vi "NA.vi"() -> ()   [LabVIEW 2020]
uses:
  <instrlib>/Agilent ENA Series/Agilent ENA Series.lvlib
panel:
  out "실수값 [dB]":dbl
  out "주파수 [MHz]":dbl
  out "읽어온 데이터":string[][](table)
  in  "s2p 저장":bool caption="빈 버튼"
  in  "파일명":string
  in  "파일명":string
  in  "저장경로":path
  in  "이미지 저장":bool caption="빈 버튼"
  in  "Reset":bool
  in  "라디오 버튼":enum32{"Center / Span", "Start / Stop"}(radio)
  in  "Stop [MHz]":dbl
  in  "Start [MHz]":dbl
  in  "Span [MHz]":dbl=2000.0
  in  "Center [MHz]":dbl=5000.0
  in  "Value Graticule Line (0.0)":dbl format="%^.2e"
  in  "Data Format":u16(ring) items=["Logarithmic Magnitude", "Phase", "Group Delay", "Smith Chart  Linear (Lin/Phase)", "Smith Chart  Logarithmic (Log/Phase)", "Smith Chart  Complex (Real/Imag)", "Smith Chart  Impedance (R+jX)", "Smith Chart  Admittance (G+jB)", "Polar Format (Linear)", "Polar Format (Logarithmic)", "Polar Format (Re/Im)", "Linear Magnitude", "SWR", "Real", "Imaginary", "Epanded Phase", "Positive Phase"]
  in  "Measurement Parameters":u16(ring)=1 items=["S11"=0, "S21"=1, "S12"=4, "S22"=5, "A"=16, "B"=17, "R1"=20, "R2"=21, "AUX1"=24, "AUX2"=25]
  in  "VISA 리소스 이름":refnum<visa-resource-name>
  in  "Hold":bool=TRUE
  out "그래프":cluster{"X":dbl, "Y":dbl}[](graph)
  in  "종료":bool
  in  "데이터 읽기":bool
  in  "설정":bool
  # "최댓값"
  # ".png"
  # ".s2p"
  # "Cont"
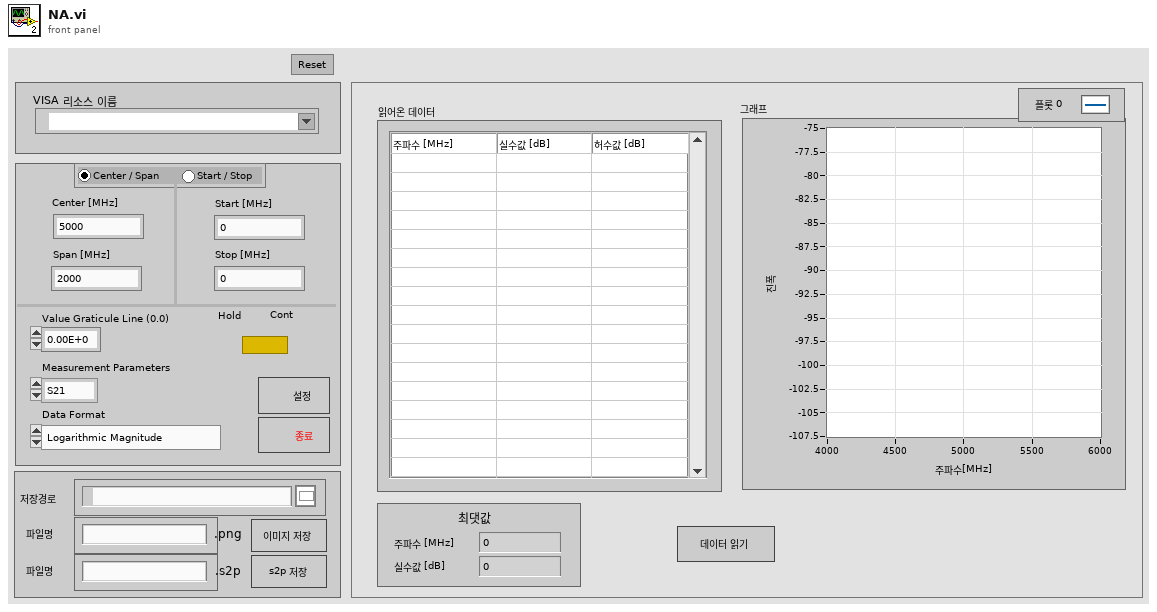
[diagram p1: front panel]
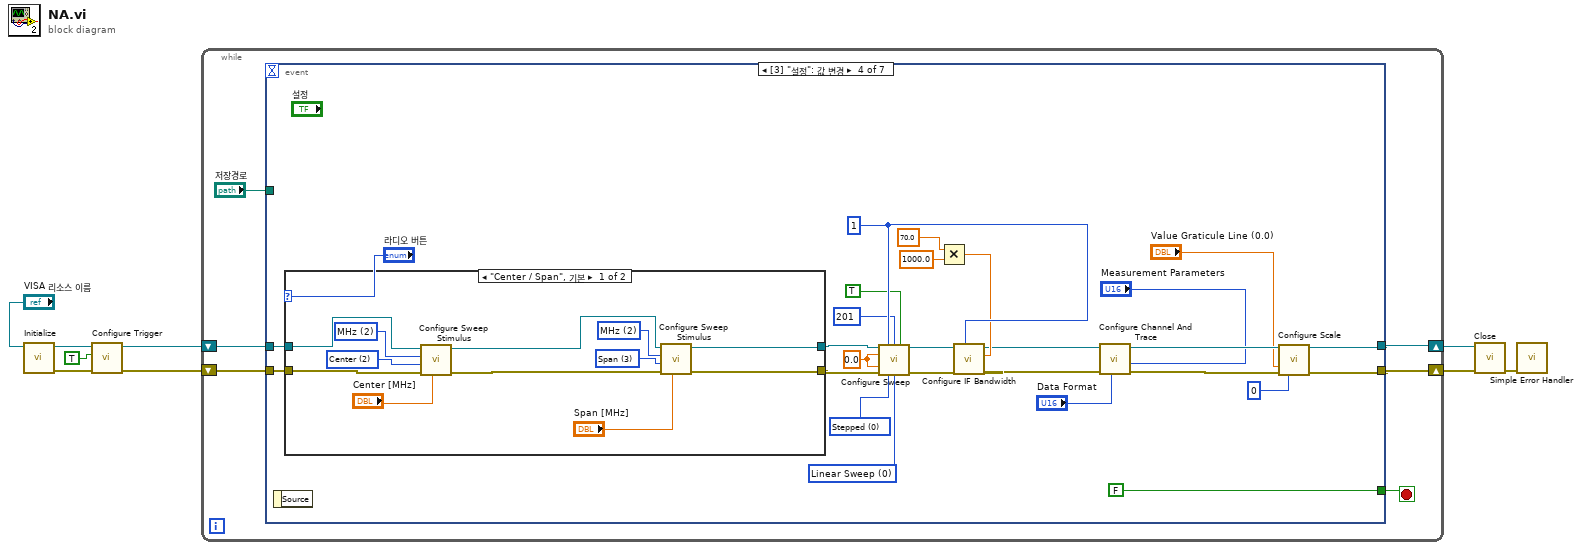
[diagram p0: block diagram]
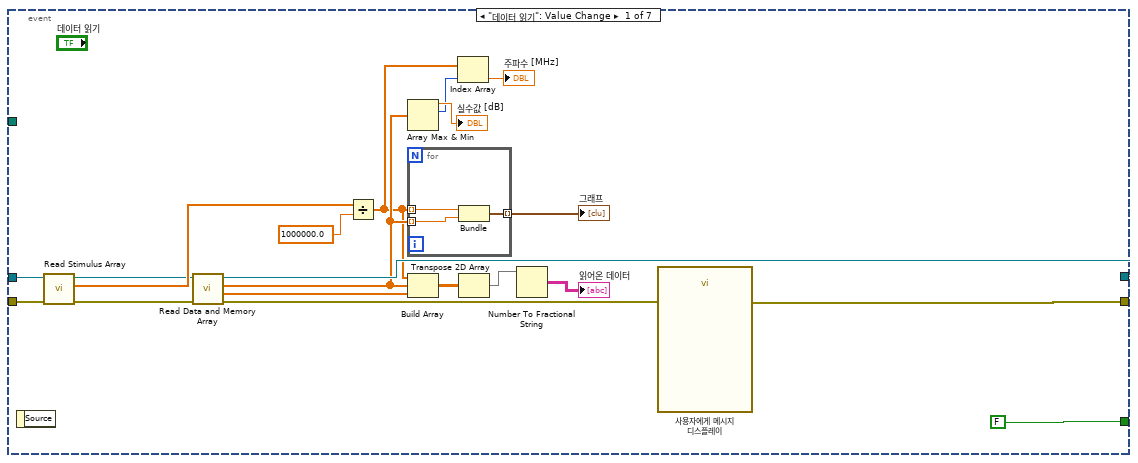
[diagram p2: hidden frame]
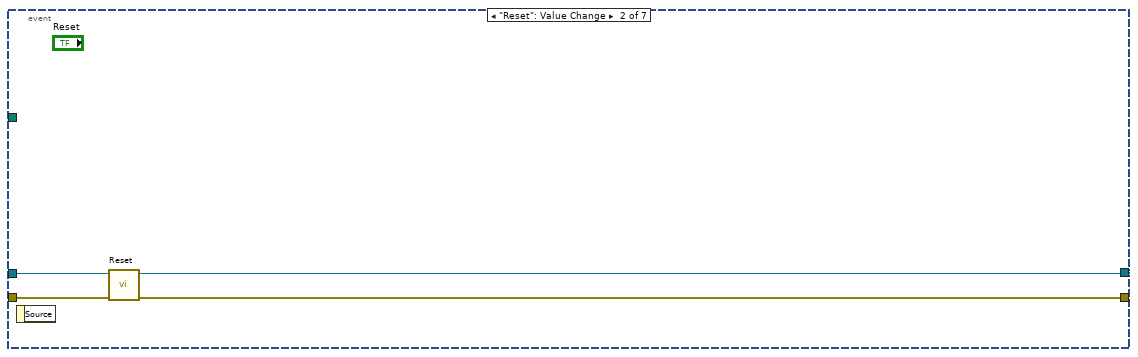
[diagram p3: hidden frame]
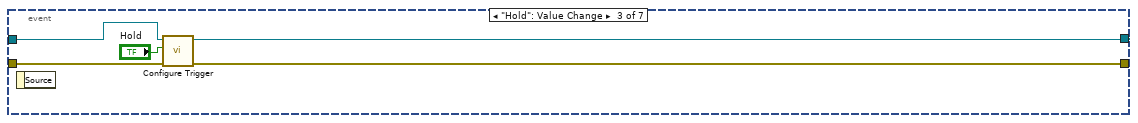
[diagram p4: hidden frame]
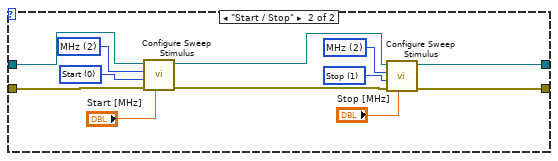
[diagram p5: hidden frame]
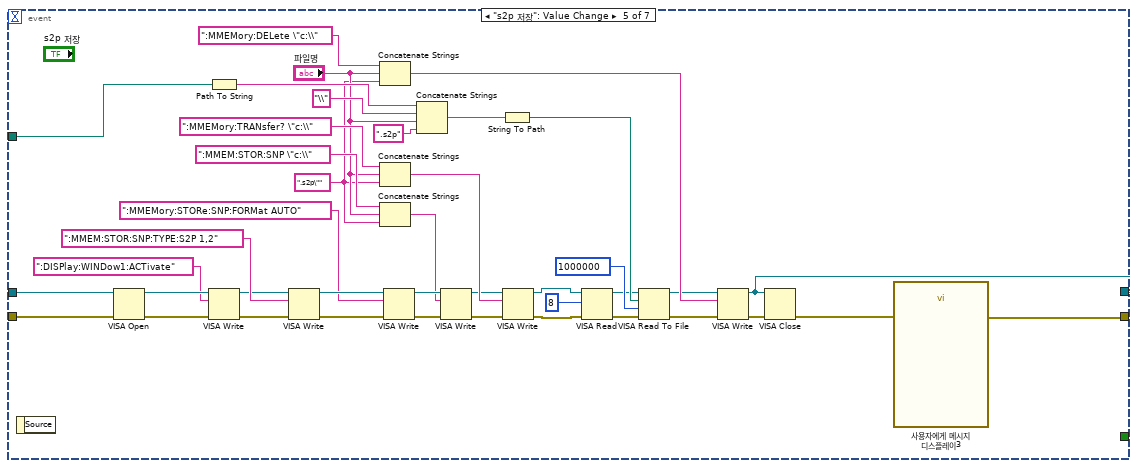
[diagram p6: hidden frame]
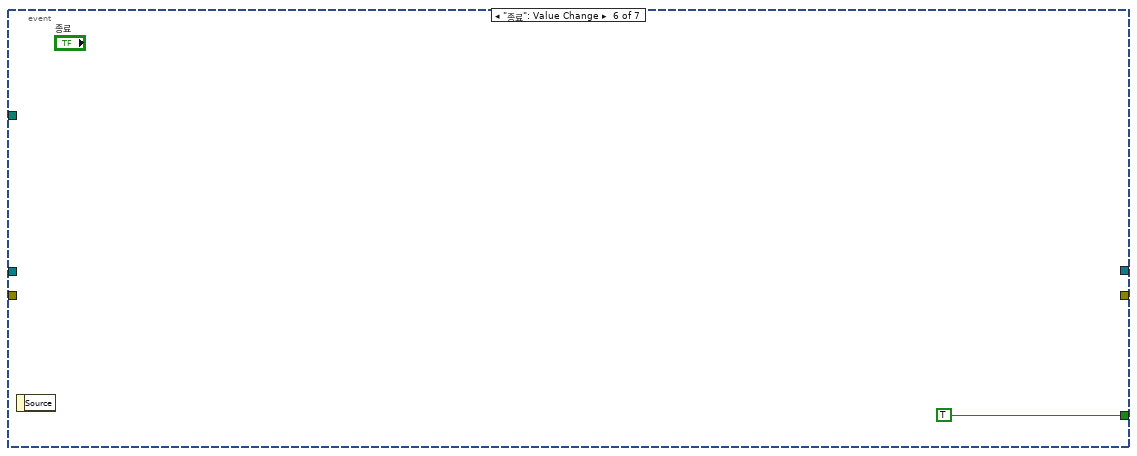
[diagram p7: hidden frame]
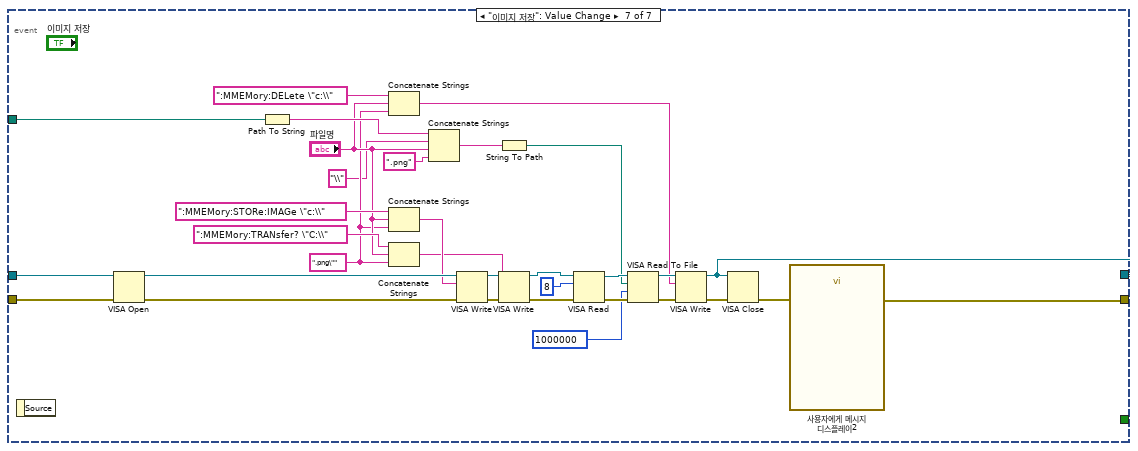
[diagram p8: hidden frame]
diagram:
  n1 = call <instrlib>:"Initialize.vi"("VISA resource name"="VISA 리소스 이름") -> ("error out"=w7:errorcluster, "VISA resource name out"=w8:refnum<visa-resource-name>)  [unwired: 9 in]
  n2 = call <instrlib>:"Configure Trigger.vi"("error in (no error)"=w7, "Continuous Sweep (T: Enable)"=TRUE, "VISA resource name"=w8) -> ("error out"=w4:errorcluster, "VISA resource name out"=w5:refnum<visa-resource-name>)  [unwired: 7 in]
  n3 = while {
    shift-right: [w13] -> w3
    shift-left: w5 -> [w15]
    shift-right: [w12] -> w2
    shift-left: w4 -> [w14]
    stop <- w10 stop-if-true
    n4 = event shown="[3] \"설정\": 값 변경" {
      selector: _ -> [_ _ _ _ _ _ _]
      dyn-events: _ -> [_ _ _ _ _ _ _]
      timeout: _ -> [_ _ _ _ _ _ _]
      tunnel: [FALSE _ _ FALSE _ TRUE _] -> w10
      tunnel: w15 -> [w29 w42 w47 w50 w120 _ w166]
      tunnel: w14 -> [w26 w41 w46 w51 w119 _ w165]
      tunnel: [w27 w40 w43 w70 w122 _ w149] -> w13
      tunnel: [w22 w39 w44 w69 w121 _ w142] -> w12
      tunnel: "저장경로" -> [_ _ _ _ w118 _ w141]
      event "데이터 읽기": Value Change {
        n5 = event-data() -> ()  [unwired: 1 in, 1 out]
        n6 = call <instrlib>:"Read Stimulus Array.vi"("error in (no error)"=w26, "VISA resource name"=w29) -> ("error out"=w25:errorcluster, "Stimulus Data"=w34:dbl[], "VISA resource name out"=w28:refnum<visa-resource-name>)  [unwired: 7 in]
        n7 = call <instrlib>:"Read Data and Memory Array.vi"("error in (no error)"=w25, "VISA resource name"=w28) -> ("error out"=w23:errorcluster, "Secondary / Imaginary"=w32:dbl[], "Primary / Real"=w20:dbl[], "VISA resource name out"=w27:refnum<visa-resource-name>)  [unwired: 6 in]
        n8 = Divide(x=w34, y=1000000.0) -> (x/y=w17:dbl[])
        n9 = Array Max & Min(array=w20) -> (max value=→"실수값 [dB]":dbl, max index (indices)=w18:i32)  [unwired: 2 out]
        n10 = for {
          tunnel: w17 -> [w38] mode=indexing
          tunnel: w20 -> [w37] mode=indexing
          tunnel: [w36] -> w24 mode=indexing
          n11 = Bundle(w38, w37) -> (w36:cluster{dbl, dbl})  [unwired: 1 in]
        }
        "그래프" <- w24
        n12 = Build Array(w17, w20, w32) -> (w31:dbl[][])
        n13 = Index Array(array=w17, index=w18) -> (element=→"주파수 [MHz]":dbl)
        n14 = Transpose 2D Array(2D array=w31) -> (transposed array=w30:dbl[][])
        n15 = Number To Fractional String(number=w30) -> (F-format string=→"읽어온 데이터":string[][])  [unwired: 3 in]
        n16 = call "사용자에게 메시지 디스플레이"("error in (no error)"=w23) -> ("error out"=w22:errorcluster)  [unwired: 9 in, 1 out]
      }
      event "Reset": Value Change {
        n17 = event-data() -> ()  [unwired: 1 in, 1 out]
        n18 = call <instrlib>:"Reset.vi"("error in (no error)"=w41, "VISA resource name"=w42) -> ("error out"=w39:errorcluster, "VISA resource name out"=w40:refnum<visa-resource-name>)  [unwired: 8 in]
      }
      event "Hold": Value Change {
        n19 = event-data() -> ()  [unwired: 1 in, 1 out]
        n20 = call <instrlib>:"Configure Trigger.vi"("error in (no error)"=w46, "Continuous Sweep (T: Enable)"="Hold", "VISA resource name"=w47) -> ("error out"=w44:errorcluster, "VISA resource name out"=w43:refnum<visa-resource-name>)  [unwired: 7 in]
      }
      event "설정": Value Change {
        w59 = 0.0 ("Sweep Time (0.001)")
        w60 = u16 0 items=["Linear Sweep", "Logarithmic Sweep", "Segment Sweep", "Power Sweep", "DC Bias"] ("Sweep Type (0: Linear Sweep)")
        w61 = u16 0 items=["Stepped", "Swept", "Fast Stepped Mode", "Fast Swept Mode"] ("Sweep Mode (0: Stepped)")
        w66 = 1 ("Channel (1)")
        n21 = event-data() -> ()  [unwired: 1 in, 1 out]
        n22 = case shown="\"Center / Span\", 기본" "라디오 버튼" {
          tunnel: [w77 w88] -> w49
          tunnel: [w78 w87] -> w48
          tunnel: w51 -> [w75 w92]
          tunnel: w50 -> [w76 w89]
          frame "Center / Span", Default {
            w82 = u16 2 items=["Hz", "kHz", "MHz", "GHz", "dBm", "s", "V"] ("Unit (0: Hz)")
            w80 = u16 2 items=["Hz", "kHz", "MHz", "GHz", "dBm", "s", "V"] ("Unit (0: Hz)")
            w83 = u16 3 items=["Start", "Stop", "Center", "Span"] ("Stimulus (0: Start)")
            w81 = u16 2 items=["Start", "Stop", "Center", "Span"] ("Stimulus (0: Start)")
            n23 = call <instrlib>:"Configure Sweep Stimulus.vi"("Parameter (0.0)"="Center [MHz]", "error in (no error)"=w75, "Stimulus (0: Start)"=w81, "Unit (0: Hz)"=w80, "VISA resource name"=w76) -> ("error out"=w84:errorcluster, "VISA resource name out"=w85:refnum<visa-resource-name>)  [unwired: 5 in]
            n24 = call <instrlib>:"Configure Sweep Stimulus.vi"("Parameter (0.0)"="Span [MHz]", "error in (no error)"=w84, "Stimulus (0: Start)"=w83, "Unit (0: Hz)"=w82, "VISA resource name"=w85) -> ("error out"=w77:errorcluster, "VISA resource name out"=w78:refnum<visa-resource-name>)  [unwired: 5 in]
          }
          frame "Start / Stop" {
            w93 = u16 2 items=["Hz", "kHz", "MHz", "GHz", "dBm", "s", "V"] ("Unit (0: Hz)")
            w94 = u16 1 items=["Start", "Stop", "Center", "Span"] ("Stimulus (0: Start)")
            w91 = u16 0 items=["Start", "Stop", "Center", "Span"] ("Stimulus (0: Start)")
            w90 = u16 2 items=["Hz", "kHz", "MHz", "GHz", "dBm", "s", "V"] ("Unit (0: Hz)")
            n25 = call <instrlib>:"Configure Sweep Stimulus.vi"("Parameter (0.0)"="Start [MHz]", "error in (no error)"=w92, "Stimulus (0: Start)"=w91, "Unit (0: Hz)"=w90, "VISA resource name"=w89) -> ("error out"=w97:errorcluster, "VISA resource name out"=w95:refnum<visa-resource-name>)  [unwired: 5 in]
            n26 = call <instrlib>:"Configure Sweep Stimulus.vi"("Parameter (0.0)"="Stop [MHz]", "error in (no error)"=w97, "Stimulus (0: Start)"=w94, "Unit (0: Hz)"=w93, "VISA resource name"=w95) -> ("error out"=w88:errorcluster, "VISA resource name out"=w87:refnum<visa-resource-name>)  [unwired: 5 in]
          }
        }
        n27 = call <instrlib>:"Configure Sweep.vi"("VISA resource name"=w48, "Channel (1)"=w66, "Number of Measurement Points (201)"=201, "Auto Sweep Time (F: Off)"=TRUE, "Sweep Time (0.001)"=w59, "Delay Time (0.001)"=w59, "error in (no error)"=w49, "Sweep Mode (0: Stepped)"=w61, "Sweep Type (0: Linear Sweep)"=w60) -> ("VISA resource name out"=w68:refnum<visa-resource-name>, "error out"=w67:errorcluster)  [unwired: 5 in]
        n28 = Multiply(x=70.0, y=1000.0) -> (x*y=w64:dbl)
        n29 = call <instrlib>:"Configure IF Bandwidth.vi"("Channel (1)"=w66, "error in (no error)"=w67, "IF Bandwidth (100000.0)"=w64, "VISA resource name"=w68) -> ("error out"=w56:errorcluster, "VISA resource name out"=w57:refnum<visa-resource-name>)  [unwired: 6 in]
        n30 = call <instrlib>:"Configure Channel And Trace.vi"("Data Format (0: Logarithmic Magnitude)"="Data Format", "error in (no error)"=w56, "Measurement Parameters (0: S11)"="Measurement Parameters", "VISA resource name"=w57) -> ("error out"=w73:errorcluster, "VISA resource name out"=w74:refnum<visa-resource-name>)  [unwired: 6 in]
        n31 = call <instrlib>:"Configure Scale.vi"("VISA resource name"=w74, "Value Graticule Line (0.0)"="Value Graticule Line (0.0)", "error in (no error)"=w73, "Reference Graticule Line (5)"=0) -> ("VISA resource name out"=w70:refnum<visa-resource-name>, "error out"=w69:errorcluster)  [unwired: 10 in]
      }
      event "s2p 저장": Value Change {
        w99 = ".s2p\"" ("문자열")
        n32 = event-data() -> ()  [unwired: 1 in, 1 out]
        n33 = VISA Open(error in (no error)=w119, VISA resource name=w120) -> (VISA resource name=w116:refnum<visa-resource-name>, error out=w115:errorcluster)  [unwired: 3 in]
        n34 = Path To String(path=w118) -> (string=w132:string)
        n35 = VISA Write(VISA resource name=w116, write buffer=":DISPlay:WINDow1:ACTivate" ("버퍼 쓰기"), error in (no error)=w115) -> (VISA resource name out=w114:refnum<visa-resource-name>, error out=w113:errorcluster)  [unwired: 1 out]
        n36 = VISA Write(VISA resource name=w114, write buffer=":MMEM:STOR:SNP:TYPE:S2P 1,2" ("버퍼 쓰기"), error in (no error)=w113) -> (VISA resource name out=w111:refnum<visa-resource-name>, error out=w110:errorcluster)  [unwired: 1 out]
        n37 = Concatenate Strings(":MMEMory:DELete \"c:\\" ("버퍼 쓰기"), "파일명", w99) -> (w137:string)
        n38 = Concatenate Strings(":MMEMory:TRANsfer? \"c:\\" ("버퍼 쓰기"), "파일명", w99) -> (w130:string)
        n39 = Concatenate Strings(":MMEM:STOR:SNP \"c:\\" ("버퍼 쓰기"), "파일명", w99) -> (w100:string)
        n40 = VISA Write(VISA resource name=w111, write buffer=":MMEMory:STORe:SNP:FORMat AUTO" ("버퍼 쓰기"), error in (no error)=w110) -> (VISA resource name out=w108:refnum<visa-resource-name>, error out=w104:errorcluster)  [unwired: 1 out]
        n41 = Concatenate Strings(w132, "\\" ("문자열"), "파일명", ".s2p" ("문자열")) -> (w133:string)
        n42 = VISA Write(VISA resource name=w108, write buffer=w100, error in (no error)=w104) -> (VISA resource name out=w107:refnum<visa-resource-name>, error out=w103:errorcluster)  [unwired: 1 out]
        n43 = String To Path(string=w133) -> (path=w134:path)
        n44 = VISA Write(VISA resource name=w107, write buffer=w130, error in (no error)=w103) -> (VISA resource name out=w105:refnum<visa-resource-name>, error out=w129:errorcluster)  [unwired: 1 out]
        n45 = VISA Read(VISA resource name=w105, byte count=u32 8 ("바이트 카운트"), error in (no error)=w129) -> (VISA resource name out=w106:refnum<visa-resource-name>, error out=w131:errorcluster)  [unwired: 2 out]
        n46 = VISA Read To File(8:w131, 9:u32 1000000 ("바이트 카운트"), 10:w134, 11:w106) -> (0:w136:errorcluster, 3:w135:refnum<visa-resource-name>)  [unwired: 1 out]
        n47 = VISA Write(VISA resource name=w135, write buffer=w137, error in (no error)=w136) -> (VISA resource name out=w122:refnum<visa-resource-name>, error out=w138:errorcluster)  [unwired: 1 out]
        n48 = VISA Close(VISA resource name=w122, error in (no error)=w138) -> (error out=w139:errorcluster)
        n49 = call "사용자에게 메시지 디스플레이3"("error in (no error)"=w139) -> ("error out"=w121:errorcluster)  [unwired: 9 in, 1 out]
      }
      event "종료": Value Change {
        n50 = event-data() -> ()  [unwired: 1 in, 1 out]
      }
      event "이미지 저장": Value Change {
        w146 = ".png\"" ("문자열")
        n51 = event-data() -> ()  [unwired: 1 in, 1 out]
        n52 = VISA Open(error in (no error)=w165, VISA resource name=w166) -> (VISA resource name=w172:refnum<visa-resource-name>, error out=w171:errorcluster)  [unwired: 3 in]
        n53 = Path To String(path=w141) -> (string=w157:string)
        n54 = Concatenate Strings(":MMEMory:DELete \"c:\\" ("버퍼 쓰기"), "파일명", w146) -> (w150:string)
        n55 = Concatenate Strings(":MMEMory:STORe:IMAGe \"c:\\" ("버퍼 쓰기"), "파일명", w146) -> (w163:string)
        n56 = Concatenate Strings(":MMEMory:TRANsfer? \"C:\\" ("버퍼 쓰기"), "파일명", w146) -> (w161:string)
        n57 = Concatenate Strings(w157, "\\" ("문자열"), "파일명", ".png" ("문자열")) -> (w156:string)
        n58 = VISA Write(VISA resource name=w172, write buffer=w163, error in (no error)=w171) -> (VISA resource name out=w170:refnum<visa-resource-name>, error out=w169:errorcluster)  [unwired: 1 out]
        n59 = String To Path(string=w156) -> (path=w155:path)
        n60 = VISA Write(VISA resource name=w170, write buffer=w161, error in (no error)=w169) -> (VISA resource name out=w168:refnum<visa-resource-name>, error out=w167:errorcluster)  [unwired: 1 out]
        n61 = VISA Read(VISA resource name=w168, byte count=u32 8 ("바이트 카운트"), error in (no error)=w167) -> (VISA resource name out=w159:refnum<visa-resource-name>, error out=w158:errorcluster)  [unwired: 2 out]
        n62 = VISA Read To File(8:w158, 9:u32 1000000 ("바이트 카운트"), 10:w155, 11:w159) -> (0:w152:errorcluster, 3:w153:refnum<visa-resource-name>)  [unwired: 1 out]
        n63 = VISA Write(VISA resource name=w153, write buffer=w150, error in (no error)=w152) -> (VISA resource name out=w149:refnum<visa-resource-name>, error out=w148:errorcluster)  [unwired: 1 out]
        n64 = VISA Close(VISA resource name=w149, error in (no error)=w148) -> (error out=w143:errorcluster)
        n65 = call "사용자에게 메시지 디스플레이2"("error in (no error)"=w143) -> ("error out"=w142:errorcluster)  [unwired: 9 in, 1 out]
      }
    }
  }
  n66 = call <instrlib>:"Close.vi"("error in (no error)"=w2, "VISA resource name"=w3) -> ("error out"=w1:errorcluster)  [unwired: 9 in]
  n67 = call <vilib>:"Simple Error Handler.vi"("error in (no error)"=w1) -> ()  [unwired: 4 in, 5 out]
